vi "initialize Session Data.vi"(0 "OBJ - Session in":refnum<class "System Log.lvclass">, 11 "error in":errorcluster) -> (4 "OBJ - Session out":refnum<class "System Log.lvclass">, 15 "error out":errorcluster)   [LabVIEW 2014, in "System Log.lvclass"]
doc: "OVERRIDE VI\nPlaceholder for decendant sessions to initialize and set their default values"
uses:
  System Log.lvclass
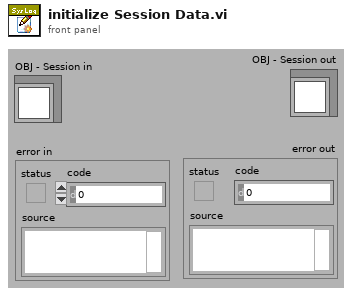
[diagram p1: front panel]
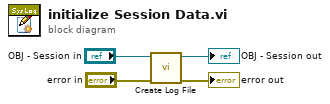
[diagram p0: block diagram]
diagram:
  n1 = call "Create Log File.vi"("error in"="error in", "Sys Log in"="OBJ - Session in") -> ("error out"=→"error out":errorcluster, "Sys Log out"=→"OBJ - Session out":refnum<class "System Log.lvclass">)  [unwired: 8 in]
